vi "scan coords to image coords.vi"(9 "scan settings":T1, 10 "tracking location":cluster{"x":i16, "y":i16, "z":i16}) -> (2 "im location":cluster{"x":i32, "y":i32, "z":i32})   [LabVIEW 2010]
uses:
  scan_specification_tagResonant.ctl
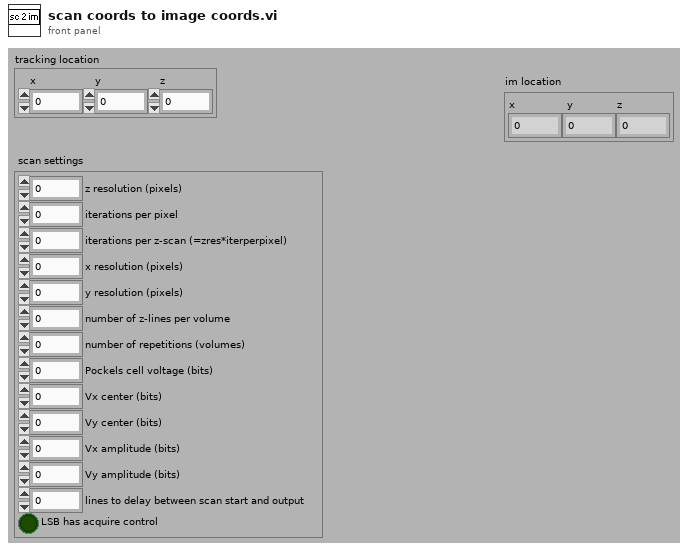
[diagram p1: front panel]
types:
  T1 = typedef "scan_specification_tagResonant.ctl" = cluster{"z resolution (pixels)":u16, "iterations per pixel":u16, "iterations per z-scan (=zres*iterperpixel)":u16, "x resolution (pixels)":u16, "y resolution (pixels)":u16, "number of z-lines per volume":u16, "number of repetitions (volumes)":i32, "Pockels cell voltage (bits)":i16, "Vx center (bits)":i16, "Vy center (bits)":i16, "Vx amplitude (bits)":i16, "Vy amplitude (bits)":i16, "lines to delay between scan start and output":u16, "LSB has acquire control":bool}
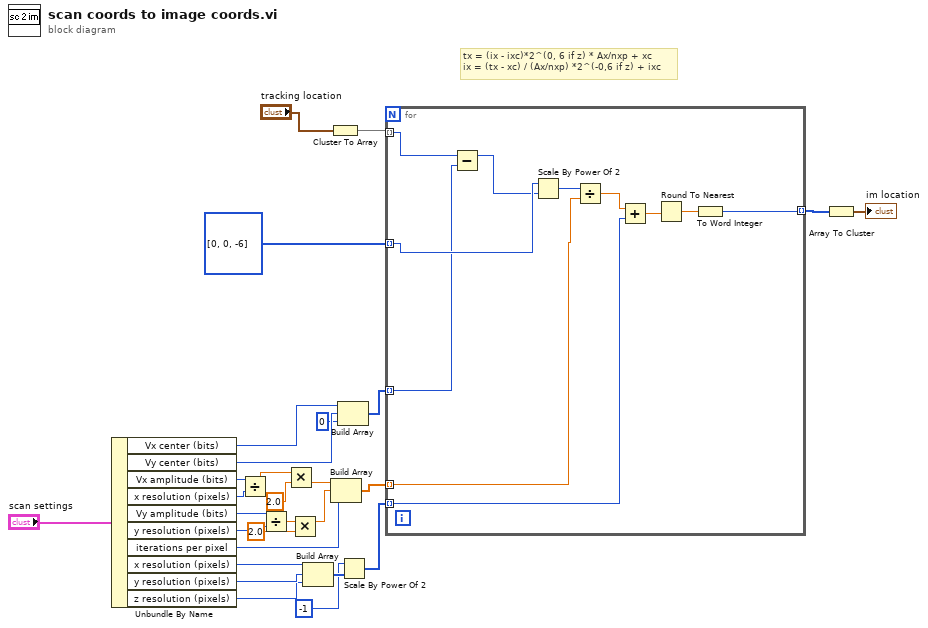
[diagram p0: block diagram]
diagram:
  # "tx = (ix - ixc)*2^(0, 6 if z) * Ax/nxp + xc\nix = (tx - xc) / (Ax/nxp) *2^(-0,6 if z) + ixc"
  n1 = Unbundle By Name("scan settings") -> ("Vx center (bits)"=w26:i16, "Vy center (bits)"=w25:i16, "Vx amplitude (bits)"=w21:i16, "x resolution (pixels)"=w22:u16, "Vy amplitude (bits)"=w20:i16, "y resolution (pixels)"=w19:u16, "iterations per pixel"=w17:u16, "x resolution (pixels)"=w15:u16, "y resolution (pixels)"=w14:u16, "z resolution (pixels)"=w13:u16)
  n2 = Divide(x=w21, y=w22) -> (x/y=w7:dbl)
  n3 = Divide(x=w20, y=w19) -> (x/y=w18:dbl)
  n4 = Multiply(x=w7, y=2.0) -> (x*y=w8:dbl)
  n5 = Multiply(x=w18, y=2.0) -> (x*y=w5:dbl)
  n6 = Build Array(w15, w14, w13) -> (w12:u16[])
  n7 = Cluster To Array(cluster="tracking location") -> (array=w3:i16[])
  n8 = Build Array(w8, w5, w17) -> (w16:dbl[])
  n9 = Build Array(w26, w25, i16 0 ("element")) -> (w23:i16[])
  n10 = Scale By Power Of 2(n=-1, x=w12) -> (x*2^n=w10:u16[])
  n11 = for {
    tunnel: i32[] [0, 0, -6] -> [w39] mode=indexing
    tunnel: w3 -> [w32] mode=indexing
    tunnel: w23 -> [w30] mode=indexing
    tunnel: w16 -> [w37] mode=indexing
    tunnel: w10 -> [w29] mode=indexing
    tunnel: [w33] -> w9 mode=indexing
    n12 = Subtract(x=w32, y=w30) -> (x-y=w31:i16)
    n13 = Scale By Power Of 2(n=w39, x=w31) -> (x*2^n=w38:i16)
    n14 = Divide(x=w38, y=w37) -> (x/y=w36:dbl)
    n15 = Add(x=w36, y=w29) -> (x+y=w35:dbl)
    n16 = Round To Nearest(number=w35) -> (nearest integer value=w34:dbl)
    n17 = To Word Integer(number=w34) -> (16bit integer=w33:i16)
  }
  n18 = Array To Cluster(array=w9) -> (cluster=→"im location":cluster{"[0]":i16, "[1]":i16, "[2]":i16})
